vi "Add Procedure_Procedure.vi"() -> ()   [LabVIEW 2019, in "Simple SysDef API.lvlib"]
uses:
  <userlib>/SimpleSysDef/Simple SysDef API.lvlib
  NationalInstruments.VeriStand.SystemDefinitionAPI
panel:
  out "error out":errorcluster
  in  "error in (no error)":errorcluster
  in  "Procedure Ref":refnum<k24>
  out "Node Ref":refnum<k24>
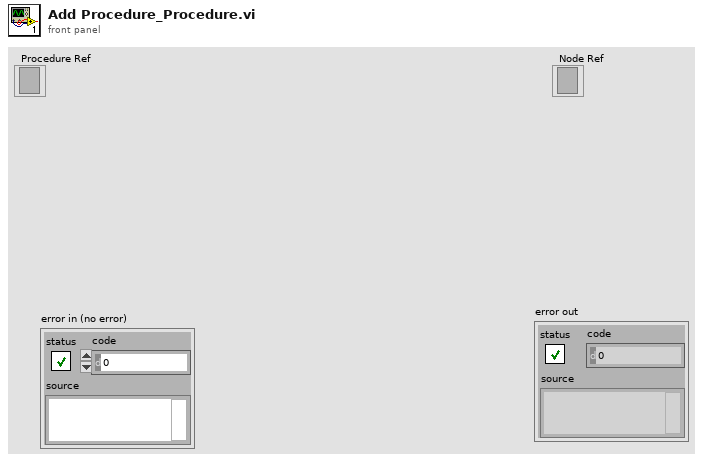
[diagram p1: front panel]
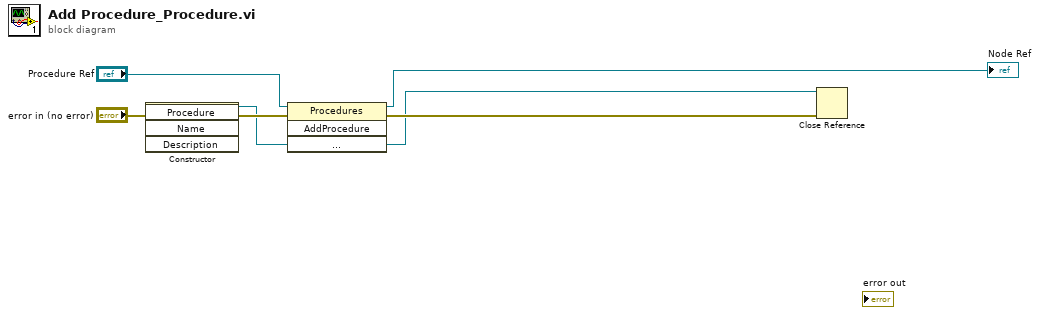
[diagram p0: block diagram]
diagram:
  n1 = constructor class="Procedure"(error in="error in (no error)") -> (reference out=w1:refnum<k24>, error out=w5:errorcluster)  [unwired: 4 in, 3 out]
  n2 = invoke class="Procedures" method="AddProcedure"(reference="Procedure Ref", error in=w5, "procedure"=w1) -> (reference out=→"Node Ref":refnum<k24>, error out=w3:errorcluster)  [unwired: 1 in, 2 out]
  n3 = Close Reference(reference=w1, error in (no error)=w3) -> ()  [unwired: 1 out]
